vi "FindSlipsFilePaths.vi"() -> (1 "Images":path, 3 "Playlists":path, 4 "Movies":path, 5 "Thumbs":path, 6 "Slides":path)   [LabVIEW 2012]
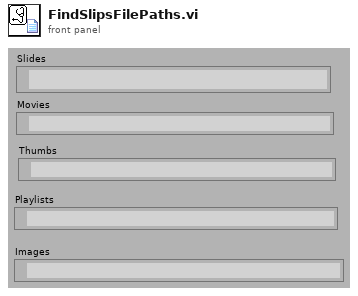
[diagram p1: front panel]
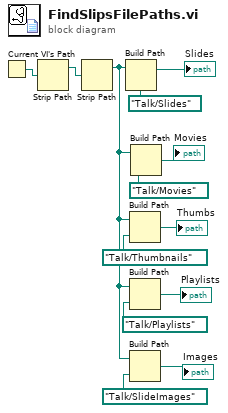
[diagram p0: block diagram]
diagram:
  n1 = Current VI's Path() -> (path=w10:path)
  n2 = Strip Path(path=w10) -> (stripped path=w11:path)  [unwired: 1 out]
  n3 = Strip Path(path=w11) -> (stripped path=w2:path)  [unwired: 1 out]
  n4 = Build Path(base path=w2, name or relative path=path "Talk/Slides" ("path to JPEG file")) -> (appended path=→"Slides":path)
  n5 = Build Path(base path=w2, name or relative path=path "Talk/Thumbnails" ("path to JPEG file")) -> (appended path=→"Thumbs":path)
  n6 = Build Path(base path=w2, name or relative path=path "Talk/Playlists" ("path to JPEG file")) -> (appended path=→"Playlists":path)
  n7 = Build Path(base path=w2, name or relative path=path "Talk/SlideImages" ("path to JPEG file")) -> (appended path=→"Images":path)
  n8 = Build Path(base path=w2, name or relative path=path "Talk/Movies" ("path to JPEG file")) -> (appended path=→"Movies":path)
